vi "warning tone.vi"(10 "Ring?":bool) -> ()   [LabVIEW 2017]
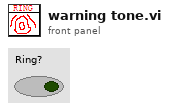
[diagram p1: front panel]
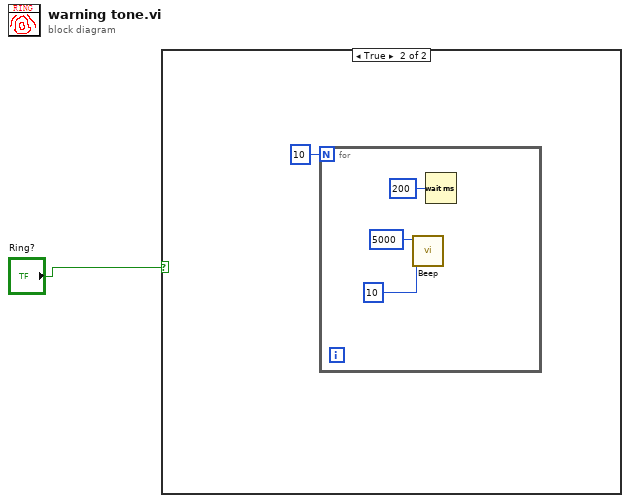
[diagram p0: block diagram]
diagram:
  n1 = case shown="True" "Ring?" {
    frame False {
    }
    frame True {
      n2 = for {
        N: 10 -> [_]
        n3 = call <vilib>:"Beep.vi"("duration (msec)"=u32 10, "frequency (Hz)"=u32 5000) -> ()  [unwired: 10 in]
        n4 = Wait (ms)(milliseconds to wait=u32 200 ("等待时间（毫秒）")) -> ()  [unwired: 1 out]
      }
    }
  }
